vi "CMD_MOVETO.vi"(6 "Gantry in":refnum<class "Gantry.lvclass">, 8 "error in (no error)":errorcluster, 10 "Arguments":string[](array[string]), 11 "gScript Interpreter in":refnum<class "gScript Interpreter.lvclass">) -> (0 "error out":errorcluster, 3 "gScript Interpreter out":refnum<class "gScript Interpreter.lvclass">, 4 "Gantry out":refnum<class "Gantry.lvclass">)   [LabVIEW 2023, in "gScript Interpreter.lvclass"]
uses:
  gScript Interpreter.lvclass
  Shared Components/Gantry Class/Gantry.lvclass
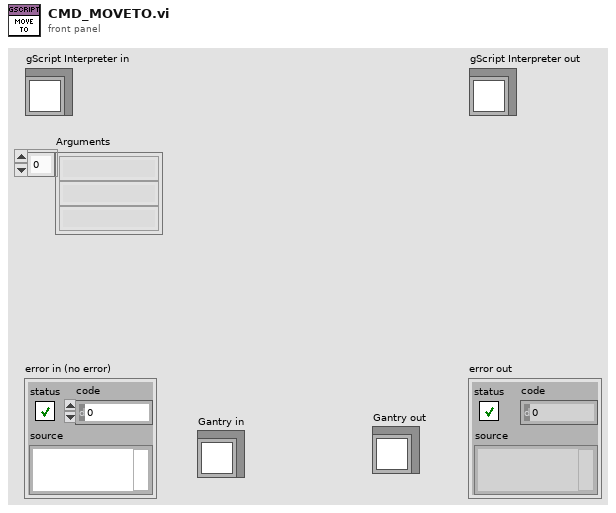
[diagram p1: front panel]
types:
  T1 = typedef "Memory Cell.ctl" = cluster{"type":T2, "x":dbl, "y":dbl, "z":dbl, "w":dbl}
  T2 = typedef "Memory Cell Type Enum.ctl" = enum16{"integer", "float", "vector", "rotation"}
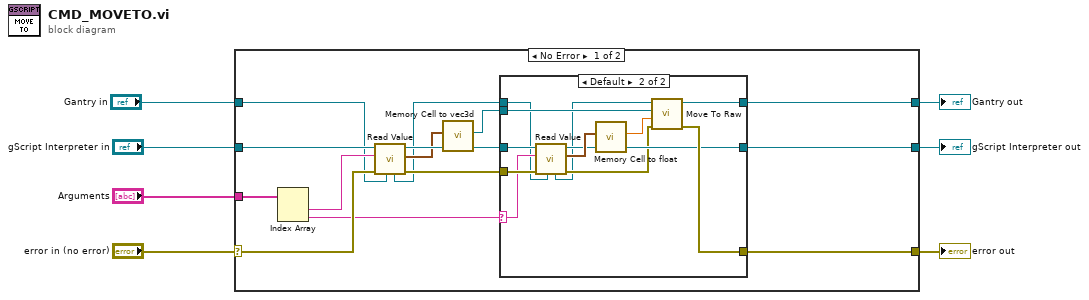
[diagram p0: block diagram]
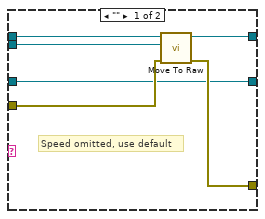
[diagram p2: hidden frame]
diagram:
  n1 = case shown="No Error" "error in (no error)" {
    selector: "error in (no error)" -> [w18 w42]
    tunnel: [w20 w42] -> w6
    tunnel: [w11 w41] -> w4
    tunnel: "gScript Interpreter in" -> [w19 w41]
    tunnel: "Arguments" -> [w17 _]
    tunnel: "Gantry in" -> [w9 w40]
    tunnel: [w21 w40] -> w1
    frame No Error {
      n2 = Index Array(array=w17) -> (element #1=w16:string, element #2=w10:string)  [unwired: 2 in]
      n3 = call-dynamic "Read Value.vi"("Gantry in"=w9, "error in (no error)"=w18, "String in"=w16, "gScript Interpreter in"=w19) -> ("error out"=w14:errorcluster, "Memory Cell"=w13:T1, "gScript Interpreter out"=w15:refnum<class "gScript Interpreter.lvclass">, "Gantry out"=w8:refnum<class "Gantry.lvclass">)  [unwired: 4 in]
      n4 = call "Memory Cell to vec3d.vi"("Memory Cell"=w13) -> ("Vec3d out"=w12:refnum<class "Vec3d.lvclass">)  [unwired: 10 in]
      n5 = case shown="Default" w10 {
        selector: w10 -> [_ w30]
        tunnel: w8 -> [w27 w29]
        tunnel: [w26 w39] -> w21
        tunnel: [w23 w38] -> w20
        tunnel: w15 -> [w22 w37]
        tunnel: w14 -> [w24 w36]
        tunnel: w12 -> [w25 w35]
        tunnel: [w22 w32] -> w11
        frame "" {
          # "Speed omitted, use default"
          n6 = call-dynamic "Move To Raw.vi"("error in"=w24, "Destination"=w25, "Gantry in"=w27) -> ("error out"=w23:errorcluster, "Gantry out"=w26:refnum<class "Gantry.lvclass">)  [unwired: 7 in]
        }
        frame Default {
          n7 = call-dynamic "Read Value.vi"("Gantry in"=w29, "error in (no error)"=w36, "String in"=w30, "gScript Interpreter in"=w37) -> ("error out"=w31:errorcluster, "Memory Cell"=w34:T1, "gScript Interpreter out"=w32:refnum<class "gScript Interpreter.lvclass">, "Gantry out"=w28:refnum<class "Gantry.lvclass">)  [unwired: 4 in]
          n8 = call "Memory Cell to float.vi"("Memory Cell"=w34) -> ("float out"=w33:dbl)  [unwired: 10 in]
          n9 = call-dynamic "Move To Raw.vi"("error in"=w31, "Speed"=w33, "Destination"=w35, "Gantry in"=w28) -> ("error out"=w38:errorcluster, "Gantry out"=w39:refnum<class "Gantry.lvclass">)  [unwired: 6 in]
        }
      }
    }
    frame Error {
    }
  }
  "error out" <- w6
  "gScript Interpreter out" <- w4
  "Gantry out" <- w1
